vi "arrayAdd.vi"(8 "error in":errorcluster, 10 "Array2":i32[](array[numeric]), 11 "Array":i32[](array[numeric])) -> (0 "error out":errorcluster, 3 "numberOut":i32[](array[numeric]))   [LabVIEW 2014]
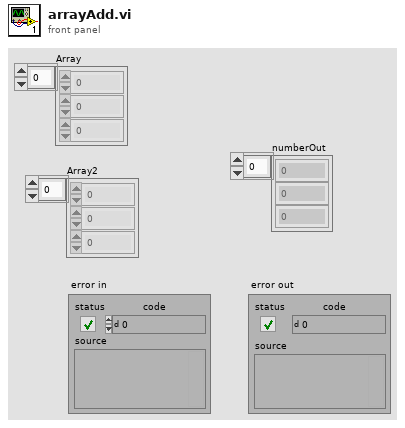
[diagram p1: front panel]
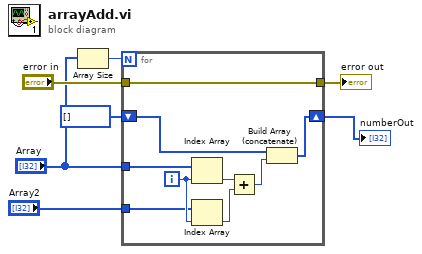
[diagram p0: block diagram]
diagram:
  n1 = Array Size(array="Array") -> (size(s)=w1:i32)
  n2 = for {
    N: w1 -> [_]
    tunnel: [w16] -> w7
    tunnel: "error in" -> [w16]
    tunnel: "Array" -> [w14]
    tunnel: "Array2" -> [w13]
    shift-right: [w9] -> w3
    shift-left: i32[] [] -> [w8]
    i -> [w15]
    n3 = Index Array(array=w14, index=w15) -> (element=w12:i32)
    n4 = Index Array(array=w13, index=w15) -> (element=w11:i32)
    n5 = Add(x=w12, y=w11) -> (x+y=w10:i32)
    n6 = Build Array (concatenate)(w8, w10) -> (w9:i32[])
  }
  "numberOut" <- w3
  "error out" <- w7
